vi "write build spec name.vi"(10 "build spec name":string, 11 "Builders in":refnum<class "Builder.lvclass">) -> (3 "Builders out":refnum<class "Builder.lvclass">)   [LabVIEW 2024, in "Builder.lvclass"]
uses:
  Builder.lvclass
  Builder.lvclass/Builder.ctl
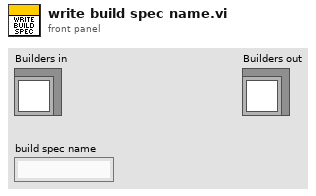
[diagram p1: front panel]
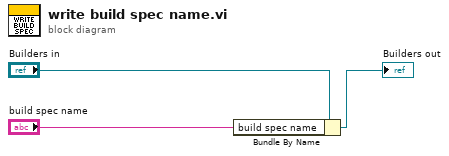
[diagram p0: block diagram]
diagram:
  n1 = Bundle By Name(cluster="Builders in", "build spec name"="build spec name") -> (→"Builders out":refnum<class "Builder.lvclass">)
